vi "formatOutputData.vi"(8 "error in (no error)":errorcluster, 11 "ILC in":refnum<class "ILC.lvclass">) -> (0 "error out":errorcluster, 2 "formattedOutputData":string, 3 "ILC out":refnum<class "ILC.lvclass">)   [LabVIEW 2015, in "ILCCommon.lvlib" / "ILC.lvclass"]
uses:
  <userlib>/Common/ILC/ILC/ILC.lvclass
  <userlib>/Common/ILC/ILC/ILC.lvclass/ILC.ctl
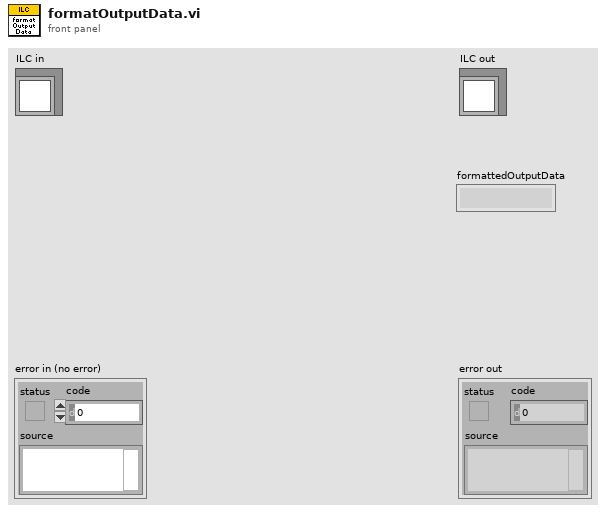
[diagram p1: front panel]
types:
  T1 = typedef "ILCCommon.lvlib/ILCTypedefs.lvlib/Outputs.ctl" = cluster{"Step & Direction":i16, "Blower RPM":u8, "PWM (SSR)":u8, "Ch1":u16, "Ch2":u16, "Ch3":u16, "Ch4":u16}
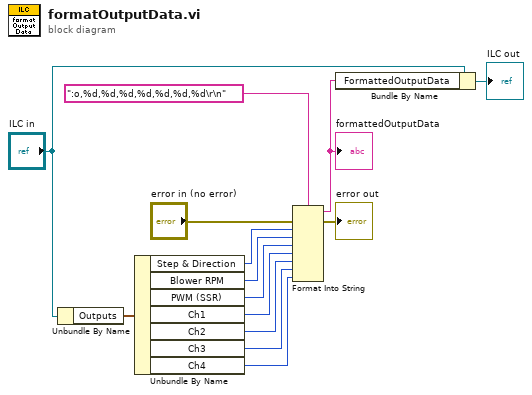
[diagram p0: block diagram]
diagram:
  n1 = Unbundle By Name("ILC in") -> ("Outputs"=w14:T1)
  n2 = Unbundle By Name(w14) -> ("Step & Direction"=w10:i16, "Blower RPM"=w9:u8, "PWM (SSR)"=w8:u8, "Ch1"=w7:u16, "Ch2"=w6:u16, "Ch3"=w5:u16, "Ch4"=w4:u16)
  n3 = Format Into String(format string=":o,%d,%d,%d,%d,%d,%d,%d\r\n", error in="error in (no error)", w10, w9, w8, w7, w6, w5, w4) -> (resulting string=w3:string, error out=→"error out":errorcluster)  [unwired: 1 in]
  "formattedOutputData" <- w3
  n4 = Bundle By Name(cluster="ILC in", "FormattedOutputData"=w3) -> (→"ILC out":refnum<class "ILC.lvclass">)
